vi "averageDownDayArrays.vi"(4 "Length":i32[](array[numeric]), 6 "Start":i32[](array[numeric]), 7 "averaging?":bool, 8 "textIn":string[][](array[string]), 9 "numericsIn":dbl[][](array[numeric]), 10 "requestedChannels":string[](array[string]), 11 "goodChannels":string[](array[string])) -> (0 "textSummary":string[][](array[string]), 1 "numericAverages":dbl[][](array[numeric]))   [LabVIEW 2022 SP3]
uses:
  <vilib>/Analysis/NI_AALBase.lvlib
  <vilib>/Analysis/baseanly.llb/Mean (DBL).vi
  b80adda9-1f56-2f48-908e-bd05a1ddb821.vi
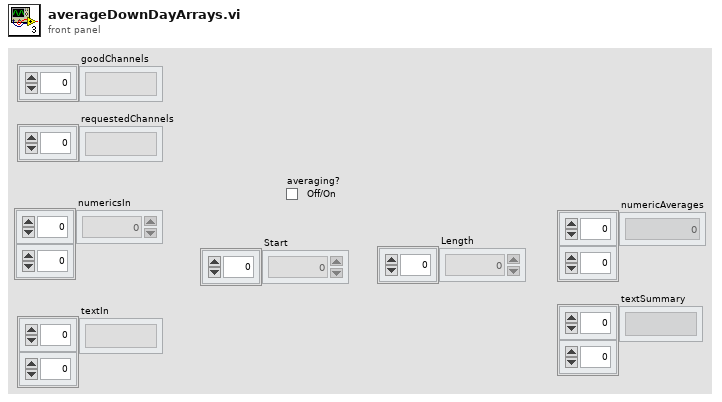
[diagram p1: front panel]
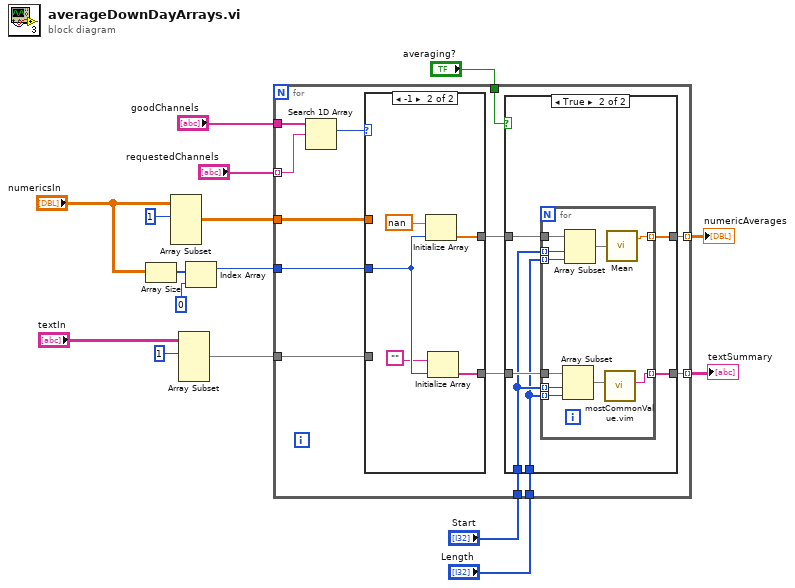
[diagram p0: block diagram]
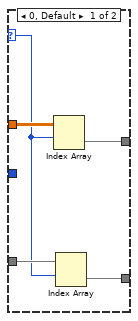
[diagram p3: hidden frame]
diagram:
  n1 = Array Size(array="numericsIn") -> (size(s)=w11:i32[])
  n2 = Array Subset(array="numericsIn", index (row)=1) -> (w9:dbl[][])  [unwired: 3 in]
  n3 = Array Subset(array="textIn", index (row)=1) -> (w2:string[][])  [unwired: 3 in]
  n4 = Index Array(array=w11, index=0 ("Index")) -> (element=w5:i32)
  n5 = for {
    tunnel: "requestedChannels" -> [w29] mode=indexing
    tunnel: "goodChannels" -> [w28]
    tunnel: w9 -> [w26]
    tunnel: [w21] -> w13 mode=indexing
    tunnel: w5 -> [w25]
    tunnel: "Start" -> [w23]
    tunnel: "Length" -> [w22]
    tunnel: "averaging?" -> [w20]
    tunnel: w2 -> [w19]
    tunnel: [w18] -> w1 mode=indexing
    n6 = Search 1D Array(1D array=w28, element=w29) -> (index of element=w27:i32)  [unwired: 1 out]
    n7 = case shown="-1" w27 {
      selector: w27 -> [w49 _]
      tunnel: w26 -> [w52 _]
      tunnel: [w51 w56] -> w24
      tunnel: w25 -> [_ w54]
      tunnel: w19 -> [w50 _]
      tunnel: [w48 w55] -> w17
      frame 0, Default {
        n8 = Index Array(array=w52, index (row)=w49) -> (element=w51:dbl[])  [unwired: 1 in]
        n9 = Index Array(array=w50, index (row)=w49) -> (element=w48:string[])  [unwired: 1 in]
      }
      frame -1 {
        n10 = Initialize Array(nan ("Number"), w54) -> (w56:dbl[])
        n11 = Initialize Array("", w54) -> (w55:string[])
      }
    }
    n12 = case shown="True" w20 {
      tunnel: w24 -> [w31 w37]
      tunnel: w23 -> [_ w34]
      tunnel: w22 -> [_ w33]
      tunnel: [w31 w36] -> w21
      tunnel: [w30 w32] -> w18
      tunnel: w17 -> [w30 w35]
      frame False {
      }
      frame True {
        n13 = for {
          tunnel: w37 -> [w47]
          tunnel: w34 -> [w46] mode=indexing
          tunnel: w33 -> [w45] mode=indexing
          tunnel: [w43] -> w36 mode=indexing
          tunnel: w35 -> [w40]
          tunnel: w34 -> [w42] mode=indexing
          tunnel: w33 -> [w41] mode=indexing
          tunnel: [w38] -> w32 mode=indexing
          n14 = Array Subset(array=w40, index=w42, length=w41) -> (w39:string[])
          n15 = Array Subset(array=w47, index=w46, length=w45) -> (w44:dbl[])
          n16 = call "mostCommonValue.vim"("arrayIn"=w39) -> ("mode"=w38:string)  [unwired: 8 in, 2 out]
          n17 = call-poly <vilib>:"Mean.vi"("X"=w44) -> ("mean"=w43:dbl)  [unwired: 1 out]
        }
      }
    }
  }
  "textSummary" <- w1
  "numericAverages" <- w13
